vi "Plugin VI.vi"(8 "error in (no error)":errorcluster, 11 "Sub Panel":refnum<vi>) -> (0 "error out":errorcluster)   [LabVIEW 2016, in "User Interface.lvlib"]
uses:
  User Interface.lvlib
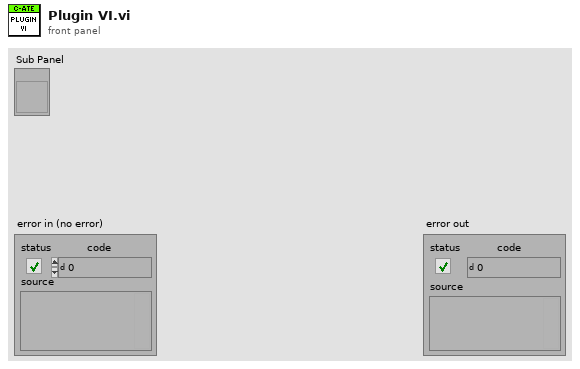
[diagram p1: front panel]
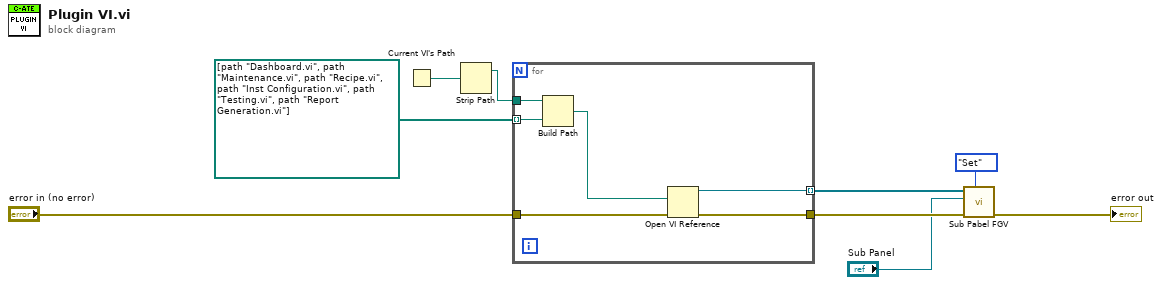
[diagram p0: block diagram]
diagram:
  n1 = Current VI's Path() -> (path=w9:path)
  n2 = Strip Path(path=w9) -> (stripped path=w8:path)  [unwired: 1 out]
  n3 = for {
    tunnel: w8 -> [w15]
    tunnel: path[] [path "Dashboard.vi", path "Maintenance.vi", path "Recipe.vi", path "Inst Configuration.vi", path "Testing.vi", path "Report Generation.vi"] -> [w14] mode=indexing
    tunnel: "error in (no error)" -> [w12]
    tunnel: [w11] -> w5
    tunnel: [w10] -> w3 mode=indexing
    n4 = Build Path(base path=w15, name or relative path=w14) -> (appended path=w13:path)
    n5 = Open VI Reference(vi path=w13, error in (no error)=w12) -> (vi reference=w10:refnum<vi>, error out=w11:errorcluster)  [unwired: 4 in]
  }
  n6 = call "Sub Pabel FGV.vi"("Command"=enum16{"Set", "Get"}."Set", "error in (no error)"=w5, "Sub Panel"="Sub Panel", "Plug in VI"=w3) -> ("error out"=→"error out":errorcluster)  [unwired: 5 in, 2 out]
